vi "DataGridViewExample.vi"() -> ()   [LabVIEW 2018]
uses:
  DataGridView_class/typedefs/ColumSetting.ctl
  DataGridView_class/typedefs/ColumnType.ctl
  DataGridView_class/DataGridView.lvclass
  System.Windows.Forms
panel:
  out "Selected Cell":string
  out "Selected Index":i32=-1
  in  "Stop":bool
  in  "DataGridView":refnum<k24>(container)
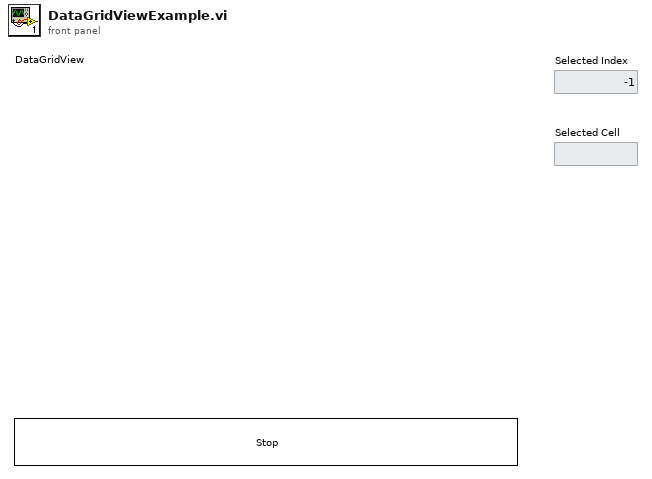
[diagram p1: front panel]
types:
  T1 = typedef "DataGridView.lvclass/ColumSetting.ctl" = cluster{"Name":string, "Datatype":T2, "Parameters":string[], "AutoSizeMode":i32, "FillWeight":sgl, "MinWidth":u32, "Width":u32, "Tooltip":string, "ReadOnly":bool}
  T2 = typedef "DataGridView.lvclass/ColumnType.ctl" = enum16{"string", "image", "check", "numeric", "timestamp", "button", "combo", "link"}
  T3 = cluster{"SelectionChangedEventReg":refnum<event-registration>, "CellClickEventReg":refnum<event-registration>}
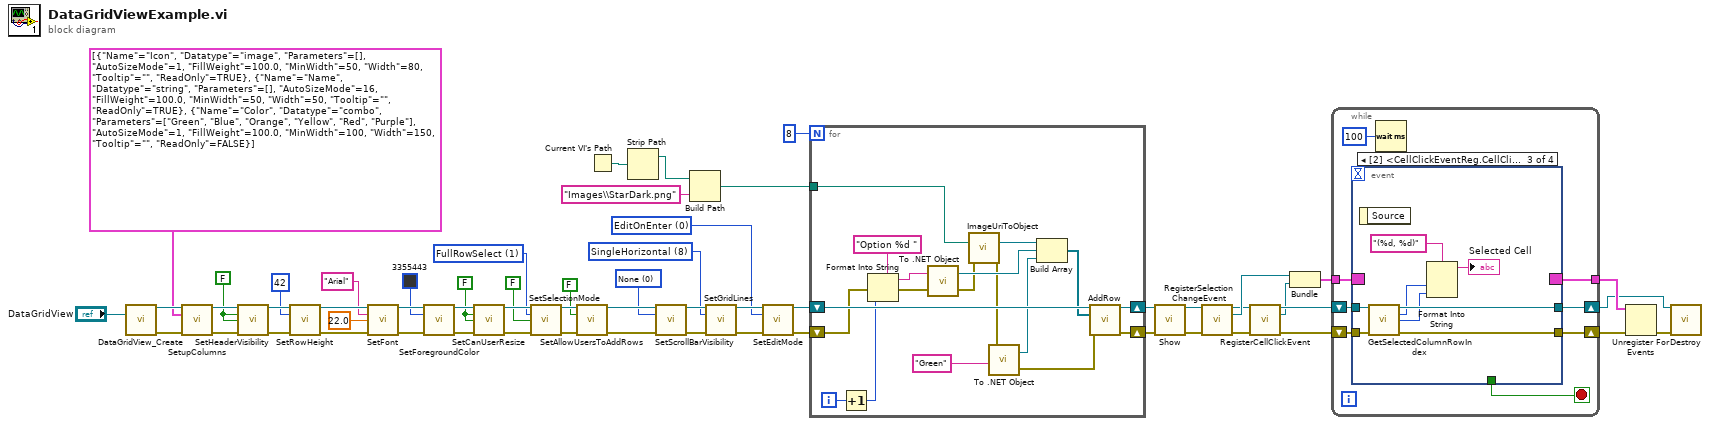
[diagram p0: block diagram]
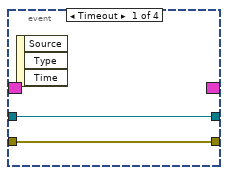
[diagram p2: hidden frame]
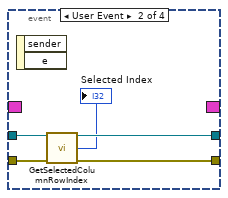
[diagram p3: hidden frame]
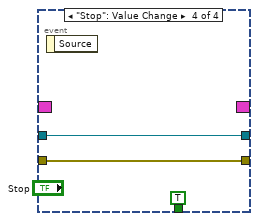
[diagram p4: hidden frame]
diagram:
  w21 = 0 items=["EditOnEnter", "EditOnKeystroke", "EditOnKeystrokeOrF2", "EditOnF2", "EditProgrammatically"] ("EditMode")
  w23 = 8 items=["Custom", "Single", "Raised", "Sunken", "None", "SingleVertical", "RaisedVertical", "SunkenVertical", "SingleHorizontal", "RaisedHorizontal", "SunkenHorizontal"] ("CellBorderStyle")
  w26 = 0 items=["None", "Horizontal", "Vertical", "Both"] ("ScrollBars")
  w33 = 1 items=["CellSelect", "FullRowSelect", "FullColumnSelect", "RowHeaderSelect", "ColumnHeaderSelect"] ("SelectionMode")
  w6 = FALSE ("ColumnHeadersVisible")
  w7 = FALSE ("ColumnHeadersVisible")
  n1 = call "DataGridView_Create.vi"("DataGridView"="DataGridView") -> ("reference out"=w54:refnum<class "DataGridView.lvclass">, "error out"=w57:errorcluster)  [unwired: 13 in]
  n2 = call-dynamic "SetupColumns.vi"("reference in"=w54, "ColumnSettings"=T1[] [{"Name"="Icon", "Datatype"=enum."image", "Parameters"=[], "AutoSizeMode"=1, "FillWeight"=100.0, "MinWidth"=50, "Width"=80, "Tooltip"="", "ReadOnly"=TRUE}, {"Name"="Name", "Datatype"=enum."string", "Parameters"=[], "AutoSizeMode"=16, "FillWeight"=100.0, "MinWidth"=50, "Width"=50, "Tooltip"="", "ReadOnly"=TRUE}, {"Name"="Color", "Datatype"=enum."combo", "Parameters"=["Green", "Blue", "Orange", "Yellow", "Red", "Purple"], "AutoSizeMode"=1, "FillWeight"=100.0, "MinWidth"=100, "Width"=150, "Tooltip"="", "ReadOnly"=FALSE}], "error in (no error)"=w57) -> ("reference out"=w47:refnum<class "DataGridView.lvclass">, "error out"=w55:errorcluster)  [unwired: 11 in]
  n3 = call-dynamic "SetHeaderVisibility.vi"("reference in"=w47, "ColumnHeadersVisible"=w7, "RowHeadersVisible"=w7, "error in (no error)"=w55) -> ("reference out"=w45:refnum<class "DataGridView.lvclass">, "error out"=w48:errorcluster)  [unwired: 10 in]
  n4 = call-dynamic "SetRowHeight.vi"("reference in"=w45, "Height"=42, "error in (no error)"=w48) -> ("reference out"=w42:refnum<class "DataGridView.lvclass">, "error out"=w46:errorcluster)  [unwired: 11 in]
  n5 = call-dynamic "SetFont.vi"("reference in"=w42, "FontName"="Arial", "emSize"=sgl 22.0, "error in (no error)"=w46) -> ("reference out"=w38:refnum<class "DataGridView.lvclass">, "error out"=w43:errorcluster)  [unwired: 10 in]
  n6 = call-dynamic "SetForegroundColor.vi"("reference in"=w38, "Color"=u32 3355443, "error in (no error)"=w43) -> ("reference out"=w18:refnum<class "DataGridView.lvclass">, "error out"=w39:errorcluster)  [unwired: 11 in]
  n7 = call-dynamic "SetCanUserResize.vi"("reference in"=w18, "AllowUserToResizeRows"=w6, "AllowUserToResizeColumns"=w6, "error in (no error)"=w39) -> ("reference out"=w34:refnum<class "DataGridView.lvclass">, "error out"=w36:errorcluster)  [unwired: 10 in]
  n8 = call-dynamic "SetSelectionMode.vi"("reference in"=w34, "SelectionMode"=w33, "MultiSelect"=FALSE, "error in (no error)"=w36) -> ("reference out"=w30:refnum<class "DataGridView.lvclass">, "error out"=w35:errorcluster)  [unwired: 10 in]
  n9 = call-dynamic "SetAllowUsersToAddRows.vi"("reference in"=w30, "AllowUserToAddRows"=FALSE, "error in (no error)"=w35) -> ("reference out"=w27:refnum<class "DataGridView.lvclass">, "error out"=w31:errorcluster)  [unwired: 11 in]
  n10 = Current VI's Path() -> (path=w10:path)
  n11 = Strip Path(path=w10) -> (stripped path=w9:path)  [unwired: 1 out]
  n12 = call-dynamic "SetScrollBarVisibility.vi"("reference in"=w27, "ScrollBars"=w26, "error in (no error)"=w31) -> ("reference out"=w24:refnum<class "DataGridView.lvclass">, "error out"=w28:errorcluster)  [unwired: 11 in]
  n13 = Build Path(base path=w9, name or relative path="Images\\StarDark.png") -> (appended path=w11:path)
  n14 = call-dynamic "SetGridLines.vi"("reference in"=w24, "CellBorderStyle"=w23, "error in (no error)"=w28) -> ("reference out"=w22:refnum<class "DataGridView.lvclass">, "error out"=w25:errorcluster)  [unwired: 11 in]
  n15 = call-dynamic "SetEditMode.vi"("reference in"=w22, "EditMode"=w21, "error in (no error)"=w25) -> ("reference out"=w19:refnum<class "DataGridView.lvclass">, "error out"=w20:errorcluster)  [unwired: 11 in]
  n16 = for {
    N: 8 -> [_]
    shift-right: [w76] -> w52
    shift-left: w20 -> [w71]
    shift-right: [w74] -> w49
    shift-left: w19 -> [w75]
    tunnel: w11 -> [w62]
    i -> [w73]
    n17 = Increment(x=w73) -> (x+1=w66:i32)
    n18 = Format Into String(format string="Option %d ", error in=w71, w66) -> (resulting string=w69:string, error out=w70:errorcluster)  [unwired: 1 in]
    n19 = call <vilib>:"To .NET Object.vi"("error in (no error)"=w70, "anything"=w69) -> ("error out"=w61:errorcluster, ".NET object"=w68:refnum<k24>)
    n20 = call "ImageUriToObject.vi"("image Path"=w62, "error in (no error)"=w61) -> (".Net Image"=w65:refnum<k24>, "error out"=w60:errorcluster)  [unwired: 12 in]
    n21 = call <vilib>:"To .NET Object.vi"("error in (no error)"=w60, "anything"="Green") -> ("error out"=w59:errorcluster, ".NET object"=w64:refnum<k24>)
    n22 = Build Array(w65, w68, w64) -> (w67:refnum<k24>[])
    n23 = call-dynamic "AddRow.vi"("reference in"=w75, "RowData"=w67, "error in (no error)"=w59) -> ("reference out"=w74:refnum<class "DataGridView.lvclass">, "error out"=w76:errorcluster)  [unwired: 11 in]
  }
  n24 = call-dynamic "Show.vi"("reference in"=w49, "error in (no error)"=w52) -> ("reference out"=w16:refnum<class "DataGridView.lvclass">, "error out"=w50:errorcluster)  [unwired: 12 in]
  n25 = call-dynamic "RegisterSelectionChangeEvent.vi"("reference in"=w16, "error in (no error)"=w50) -> ("reference out"=w3:refnum<class "DataGridView.lvclass">, "SelectionChangedEventReg"=w8:refnum<event-registration>, "error out"=w17:errorcluster)  [unwired: 11 in]
  n26 = call-dynamic "RegisterCellClickEvent.vi"("reference in"=w3, "error in (no error)"=w17) -> ("reference out"=w2:refnum<class "DataGridView.lvclass">, "CellClickEventReg"=w1:refnum<event-registration>, "error out"=w4:errorcluster)  [unwired: 11 in]
  n27 = Bundle("SelectionChangedEventReg"=w8, "CellClickEventReg"=w1) -> (w5:T3)  [unwired: 1 in]
  n28 = while {
    tunnel: w5 -> [w80]
    tunnel: [w79] -> w14
    shift-right: [w81] -> w13
    shift-left: w2 -> [w82]
    shift-right: [w78] -> w51
    shift-left: w4 -> [w84]
    stop <- w77 stop-if-true
    n29 = event shown="[2] <CellClickEventReg.CellClickEvent>: User Event" {
      selector: w80 -> [_ _ _ _]
      dyn-events: [_ _ _ _] -> w79
      timeout: _ -> [_ _ _ _]
      tunnel: w84 -> [w86 w91 w99 w101]
      tunnel: [w86 w90 w98 w101] -> w78
      tunnel: w82 -> [w85 w89 w97 w100]
      tunnel: [w85 w88 w96 w100] -> w81
      tunnel: [_ _ _ TRUE] -> w77
      event Timeout {
        n30 = event-data() -> ()  [unwired: 1 in, 3 out]
      }
      event User Event {
        n31 = event-data() -> ()  [unwired: 1 in, 2 out]
        n32 = call-dynamic "GetSelectedColumnRowIndex.vi"("reference in"=w89, "error in (no error)"=w91) -> ("reference out"=w88:refnum<class "DataGridView.lvclass">, "RowIndex"=→"Selected Index":i32, "error out"=w90:errorcluster)  [unwired: 10 in, 1 out]
      }
      event User Event {
        n33 = event-data() -> ()  [unwired: 1 in, 1 out]
        n34 = call-dynamic "GetSelectedColumnRowIndex.vi"("reference in"=w97, "error in (no error)"=w99) -> ("reference out"=w96:refnum<class "DataGridView.lvclass">, "ColumnIndex"=w93:i32, "RowIndex"=w92:i32, "error out"=w98:errorcluster)  [unwired: 10 in]
        n35 = Format Into String(format string="(%d, %d)", w93, w92) -> (resulting string=→"Selected Cell":string)  [unwired: 2 in, 1 out]
      }
      event "Stop": Value Change {
        n36 = event-data() -> ()  [unwired: 1 in, 1 out]
      }
    }
    n37 = Wait (ms)(milliseconds to wait=u32 100) -> ()  [unwired: 1 out]
  }
  n38 = Unregister For Events(event registration refnum=w14, error in=w51) -> (error out=w15:errorcluster)
  n39 = call-dynamic "Destroy.vi"("reference in"=w13, "error in (no error)"=w15) -> ()  [unwired: 12 in, 2 out]
